vi "Test Reference Channel.vi"(8 "error in (no error)":errorcluster, 11 "SR7270 Drivers in":refnum<class "SR7270 Drivers.lvclass">) -> (0 "error out":errorcluster, 3 "SR7270 Drivers out":refnum<class "SR7270 Drivers.lvclass">)   [LabVIEW 2016, in "SR7270 Drivers.lvclass"]
uses:
  SR7270 Drivers.lvclass
  <vilib>/addons/_JKI Toolkits/Caraya/classes/Test/Test.lvclass
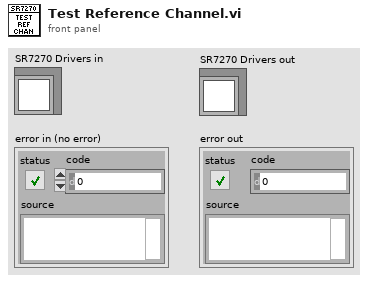
[diagram p1: front panel]
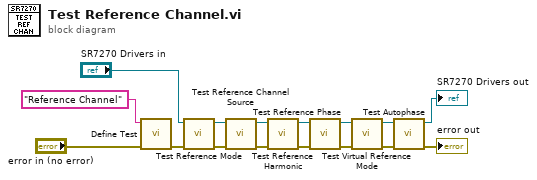
[diagram p0: block diagram]
diagram:
  n1 = call <vilib>:"Define Test.vi"("error in (no error)"="error in (no error)", "Label (VI Title)"="Reference Channel") -> ("error out"=w14:errorcluster)  [unwired: 9 in]
  n2 = call "Test Reference Mode.vi"("error in (no error)"=w14, "SR7270 Drivers in"="SR7270 Drivers in") -> ("error out"=w12:errorcluster, "SR7270 Drivers out"=w13:refnum<class "SR7270 Drivers.lvclass">)  [unwired: 8 in]
  n3 = call "Test Reference Channel Source.vi"("error in (no error)"=w12, "SR7270 Drivers in"=w13) -> ("error out"=w10:errorcluster, "SR7270 Drivers out"=w11:refnum<class "SR7270 Drivers.lvclass">)  [unwired: 8 in]
  n4 = call "Test Reference Harmonic.vi"("error in (no error)"=w10, "SR7270 Drivers in"=w11) -> ("error out"=w8:errorcluster, "SR7270 Drivers out"=w9:refnum<class "SR7270 Drivers.lvclass">)  [unwired: 8 in]
  n5 = call "Test Reference Phase.vi"("error in (no error)"=w8, "SR7270 Drivers in"=w9) -> ("error out"=w6:errorcluster, "SR7270 Drivers out"=w7:refnum<class "SR7270 Drivers.lvclass">)  [unwired: 8 in]
  n6 = call "Test Virtual Reference Mode.vi"("error in (no error)"=w6, "SR7270 Drivers in"=w7) -> ("error out"=w3:errorcluster, "SR7270 Drivers out"=w4:refnum<class "SR7270 Drivers.lvclass">)  [unwired: 8 in]
  n7 = call "Test Autophase.vi"("error in (no error)"=w3, "SR7270 Drivers in"=w4) -> ("error out"=→"error out":errorcluster, "SR7270 Drivers out"=→"SR7270 Drivers out":refnum<class "SR7270 Drivers.lvclass">)  [unwired: 8 in]
